vi "Limit Row.vi"(8 "error in (no error)":errorcluster, 10 "Limit File Path":path, 11 "Test Case":string) -> (0 "error out":errorcluster)   [LabVIEW 2024]
doc: "Vi used by the limits configurator to build the limit data."
uses:
  Step Type.ctl
  Numeric Comparison Type.ctl
  String Comparison Type.ctl
  <vilib>/addons/_JKI Toolkits/State Machine/_JKI_lib_State_Machine.llb/Periodic Trigger__ogtk__JKI-SM__jki_lib_state_machine.vi
  <vilib>/addons/_JKI Toolkits/State Machine/_JKI_lib_State_Machine.llb/Select State(s)_err__jki_lib_state_machine.vi
  <vilib>/Utility/file.llb/Read Delimited Spreadsheet (string).vi
  <userlib>/_OpenG.lib/appcontrol/appcontrol.llb/openg_application_control.lvlib
  <vilib>/Utility/file.llb/Write Delimited Spreadsheet (string).vi
panel:
  in  "Comment":string
  in  "Tab Type":enum32{"Numeric", "String", "Boolean", "Action"}(tab)
  in  "Higher Limit":string
  in  "Lower Limit":string
  in  "Numeric Comparison Type":T1 caption="Comparison Type"
  in  "String Comparison Type":T2 caption="Comparison Type"
  in  "Compare String":string
  in  "Boolean Comparison Type":T2 caption="Comparison Type"
  in  "Compare Logic":string(combo)
  out "Title Indicator":string
  in  "Cancel Button":bool
  in  "Add Button":bool
  in  "Step Type":T3
  in  "SubTest Name":string
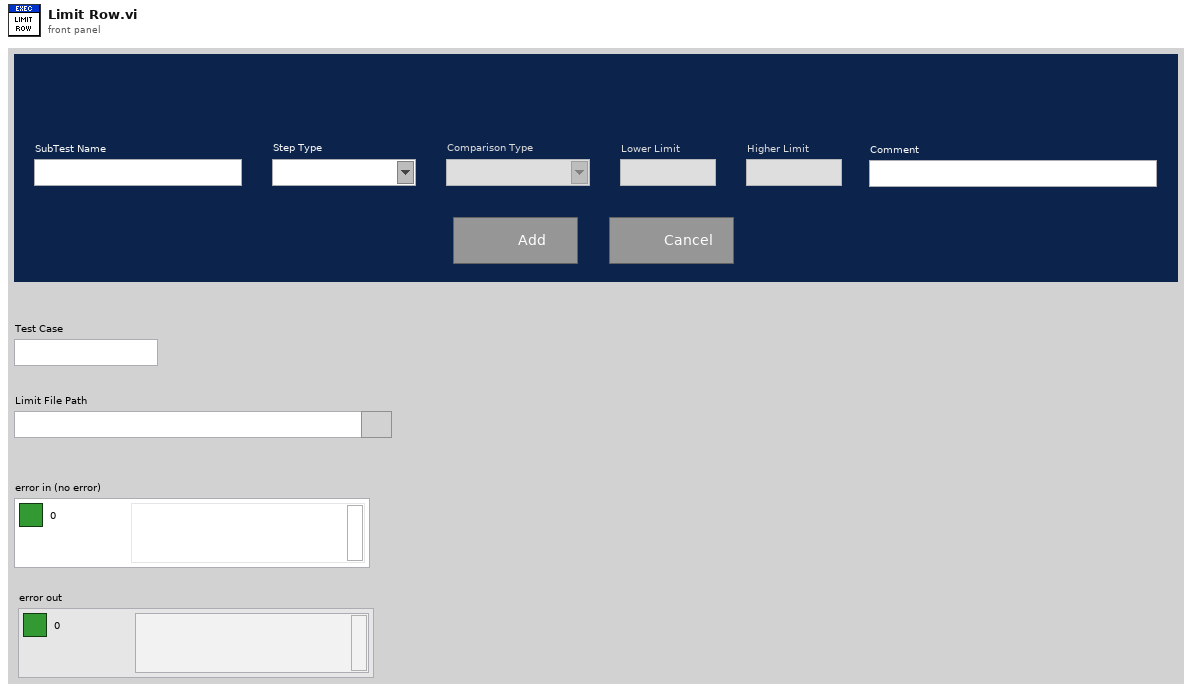
[diagram p1: front panel]
types:
  T1 = typedef "Numeric Comparison Type.ctl" = string
  T2 = typedef "String Comparison Type.ctl" = string
  T3 = typedef "Step Type.ctl" = string
  T4 = enum32{"Invalid", "Standard", "Closed", "Hidden", "Minimized", "Maximized"}
  T5 = enum32{"invalid app kind", "Development System", "Run Time System", "Student Edition", "Embedded LabVIEW", "Evaluation", "Custom"}
  T6 = enum8{"Enabled", "Disabled", "Disabled and Grayed Out"}
  T7 = cluster{"Core":cluster{"Current VI Reference":refnum<vi>, "Close Panel on Exit?":bool}, "Limit Row Array":string[], "Limit File Array":string[][], "Limit File Path":path, "Test Case":string}
  T8 = cluster{"Current VI Reference":refnum<vi>, "Close Panel on Exit?":bool}
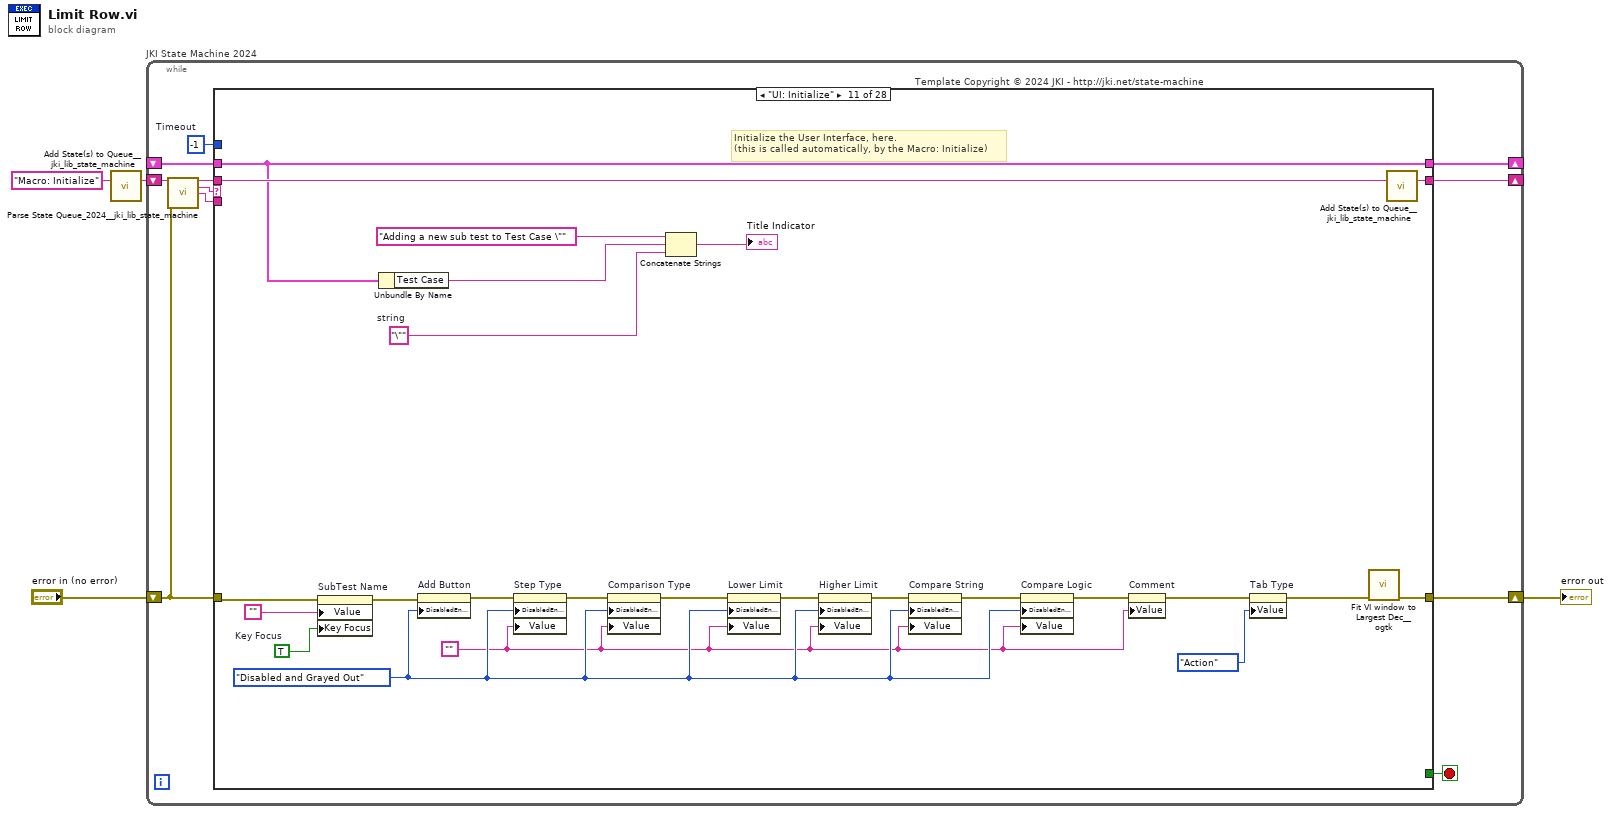
[diagram p0: block diagram]
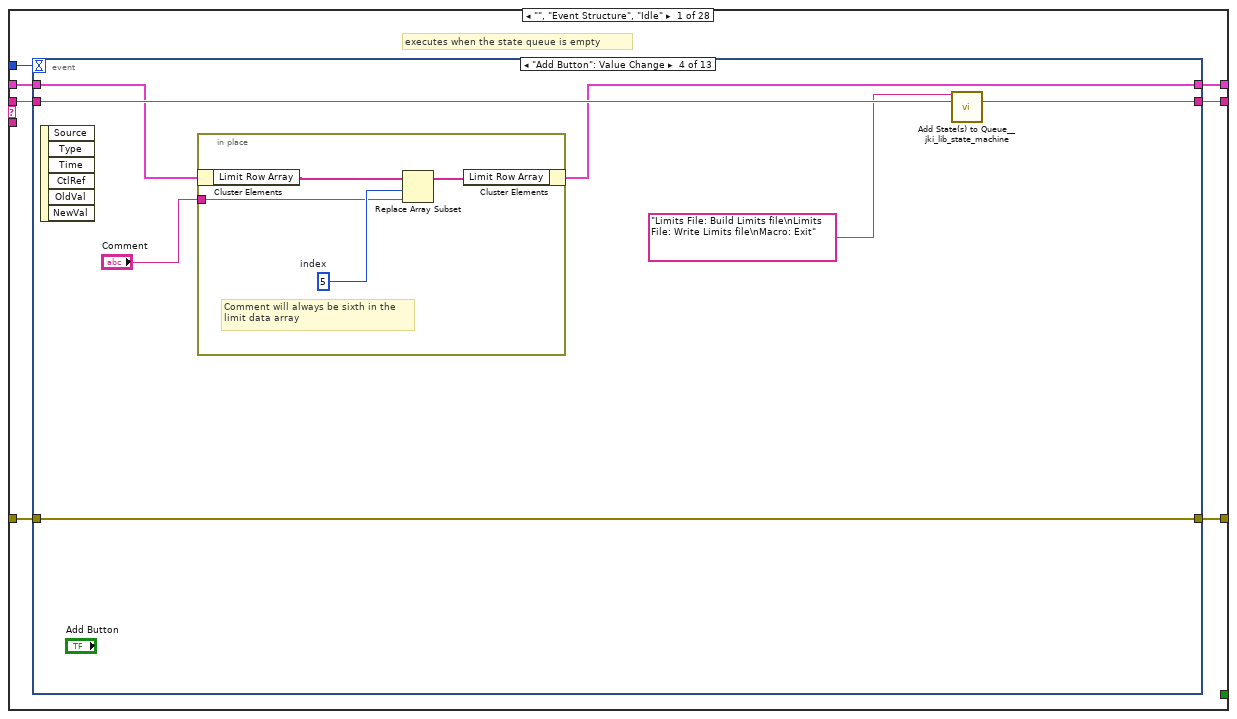
[diagram p2: hidden frame]
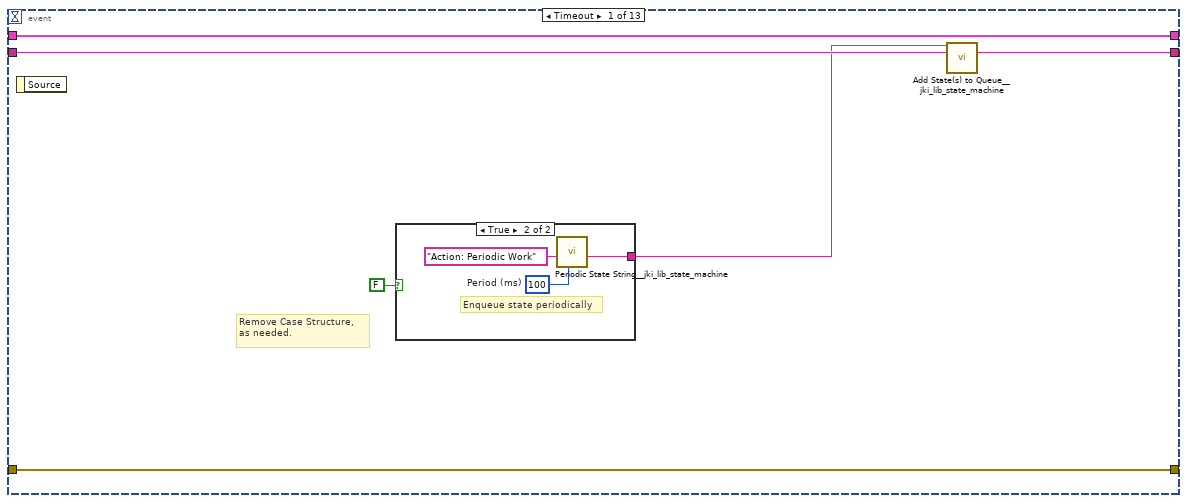
[diagram p3: hidden frame]
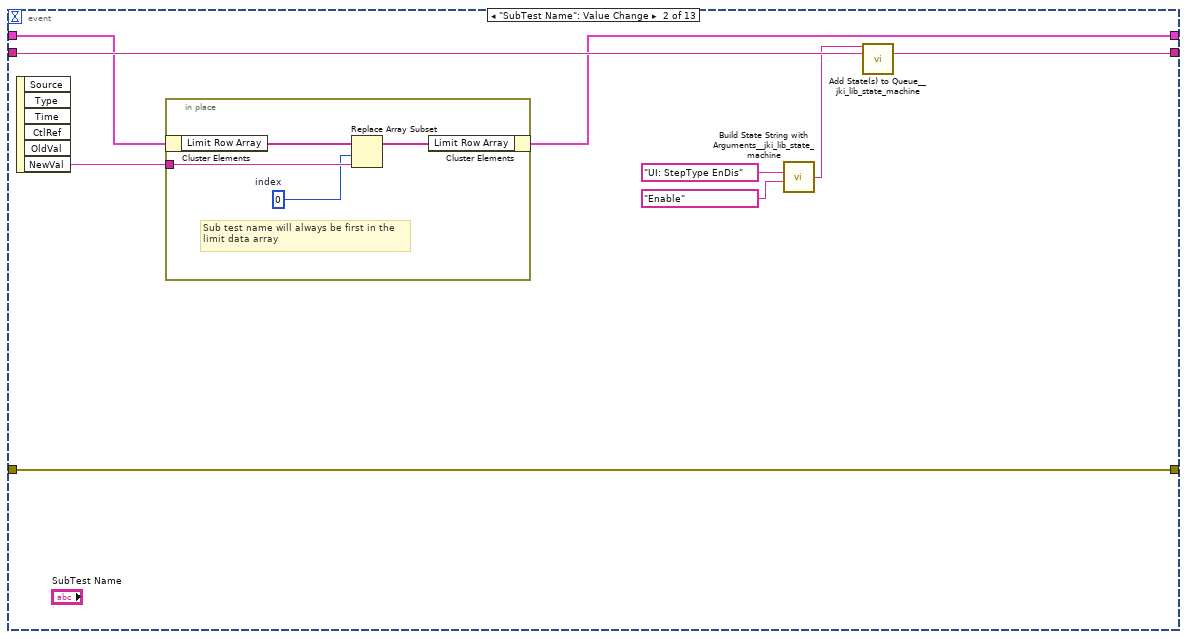
[diagram p5: hidden frame]
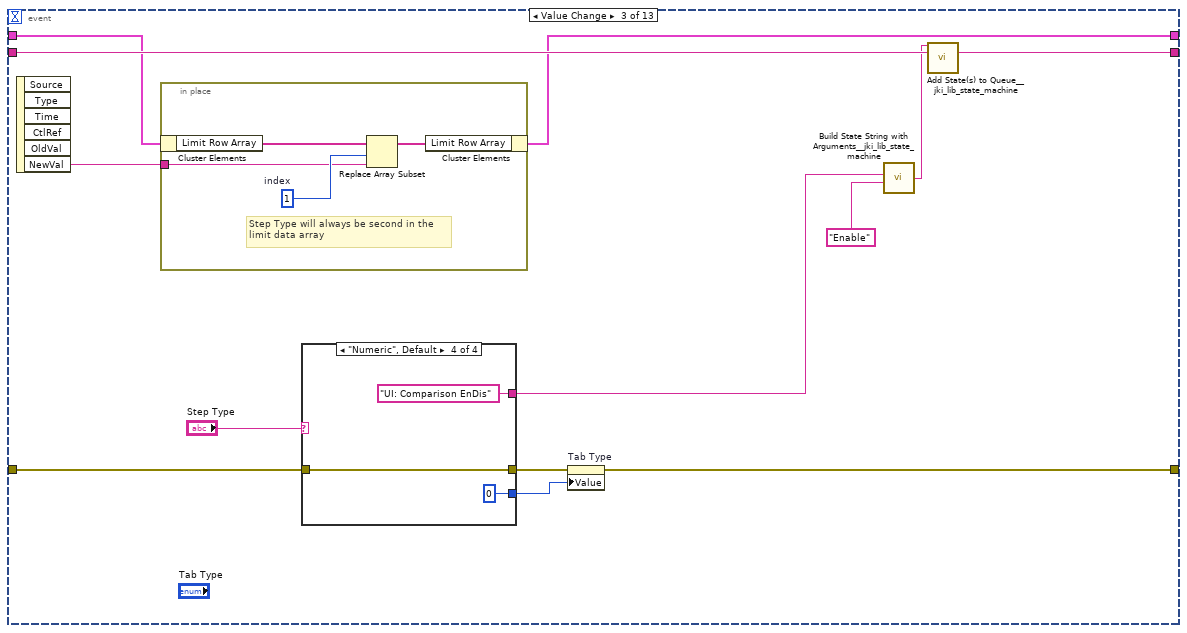
[diagram p6: hidden frame]
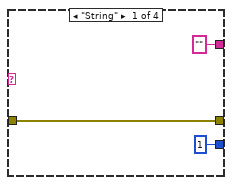
[diagram p7: hidden frame]
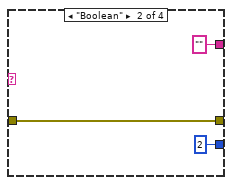
[diagram p8: hidden frame]
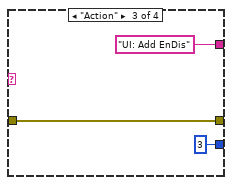
[diagram p9: hidden frame]
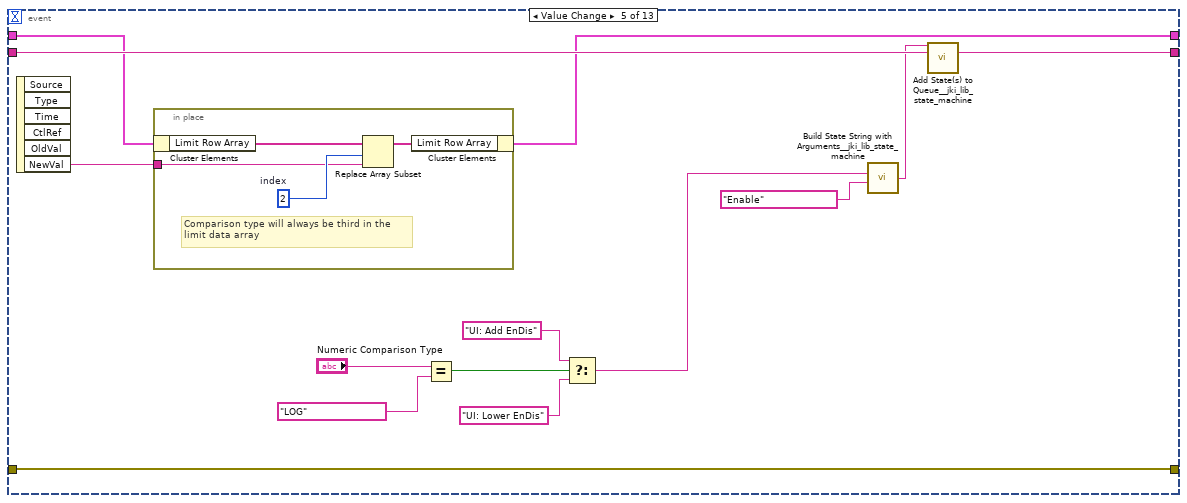
[diagram p10: hidden frame]
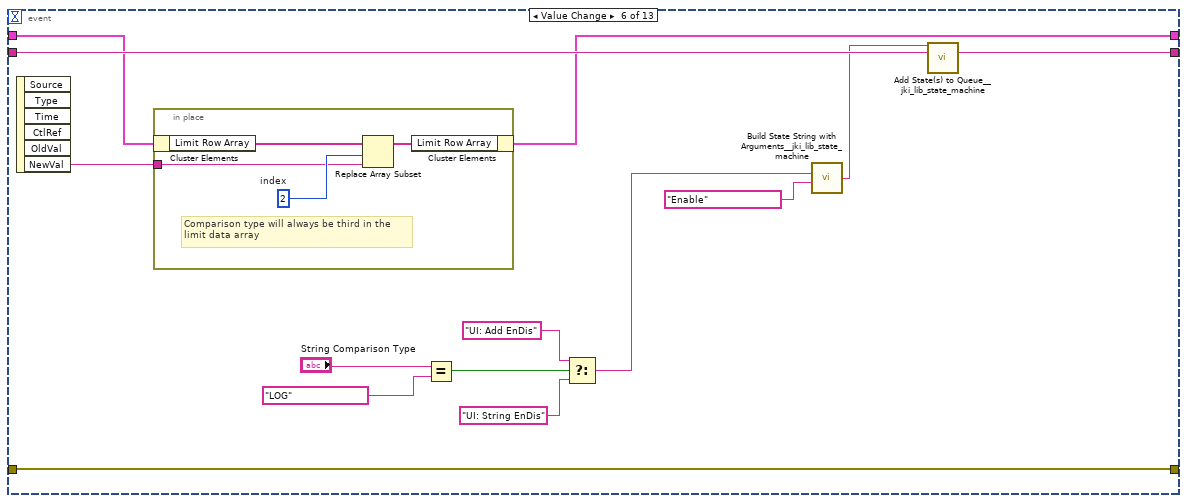
[diagram p11: hidden frame]
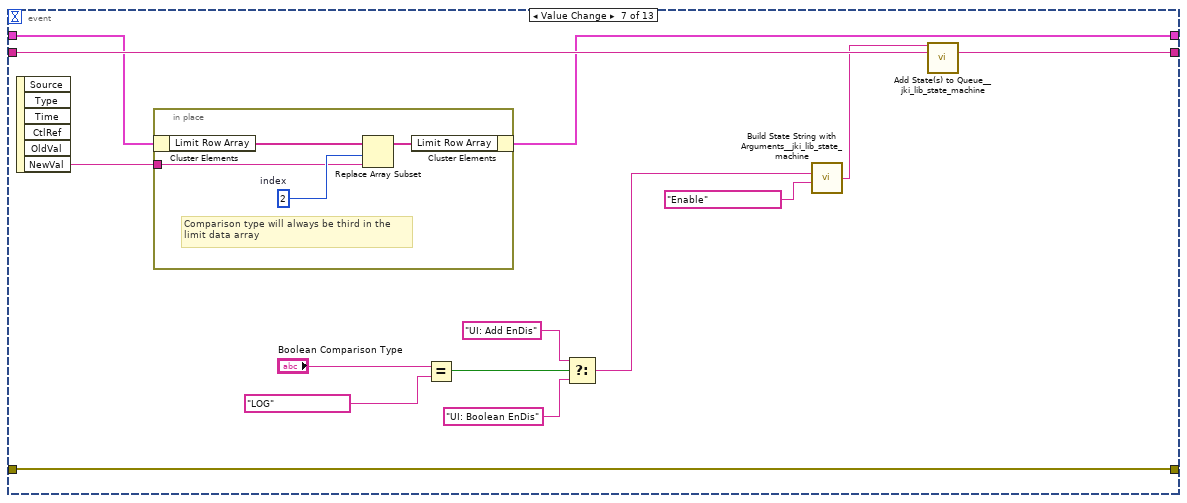
[diagram p12: hidden frame]
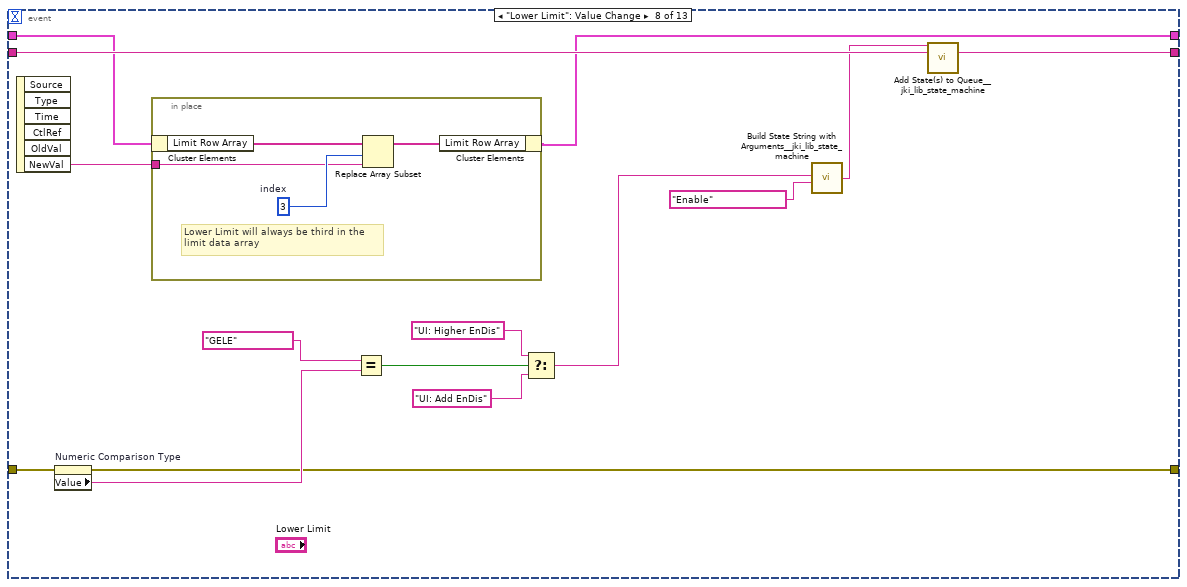
[diagram p13: hidden frame]
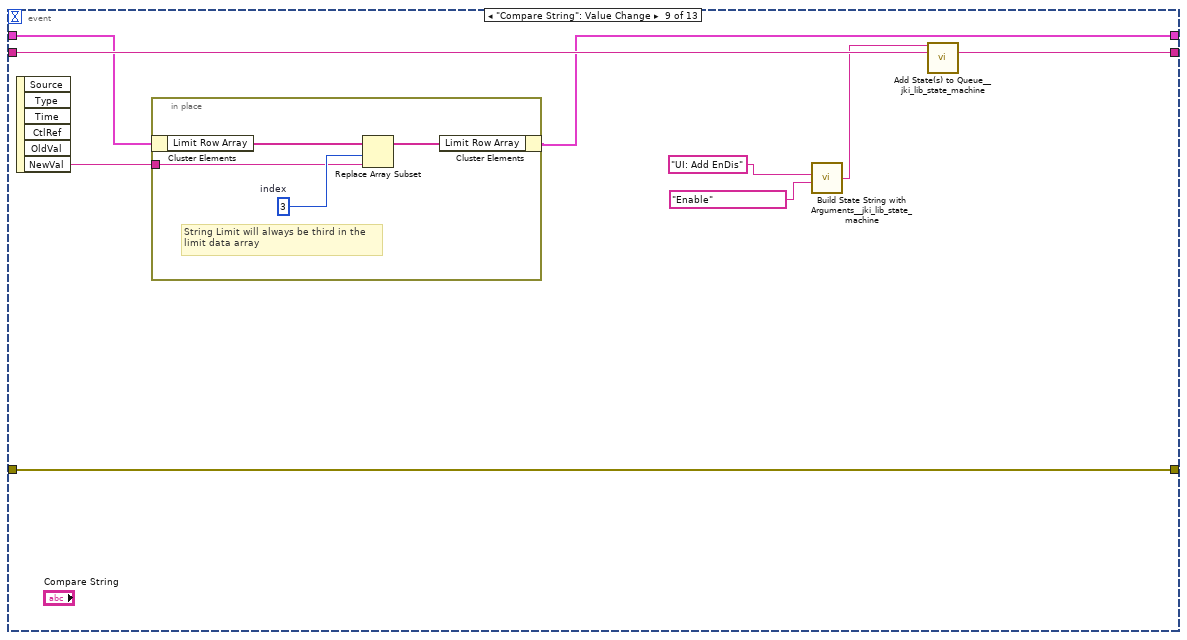
[diagram p14: hidden frame]
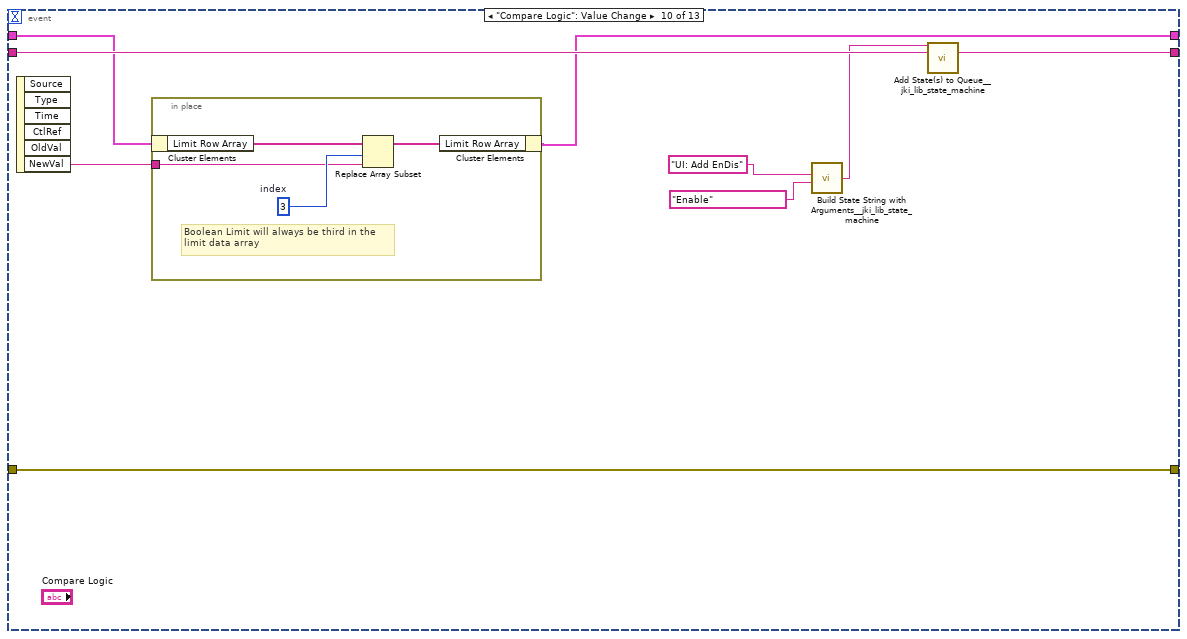
[diagram p15: hidden frame]
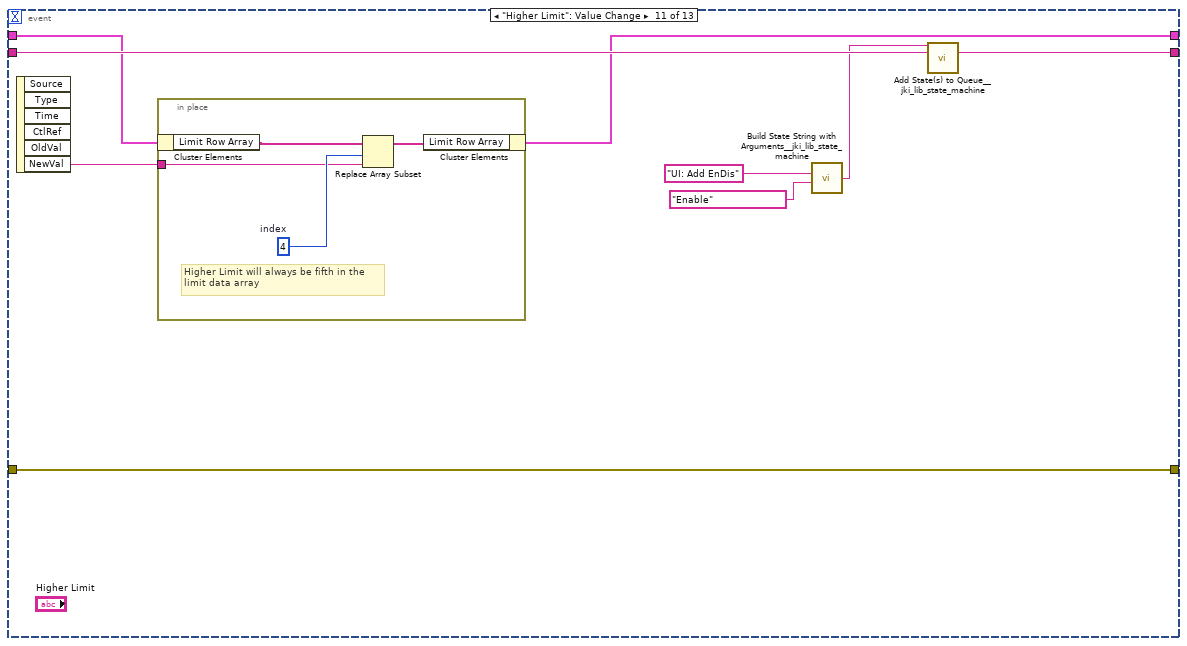
[diagram p16: hidden frame]
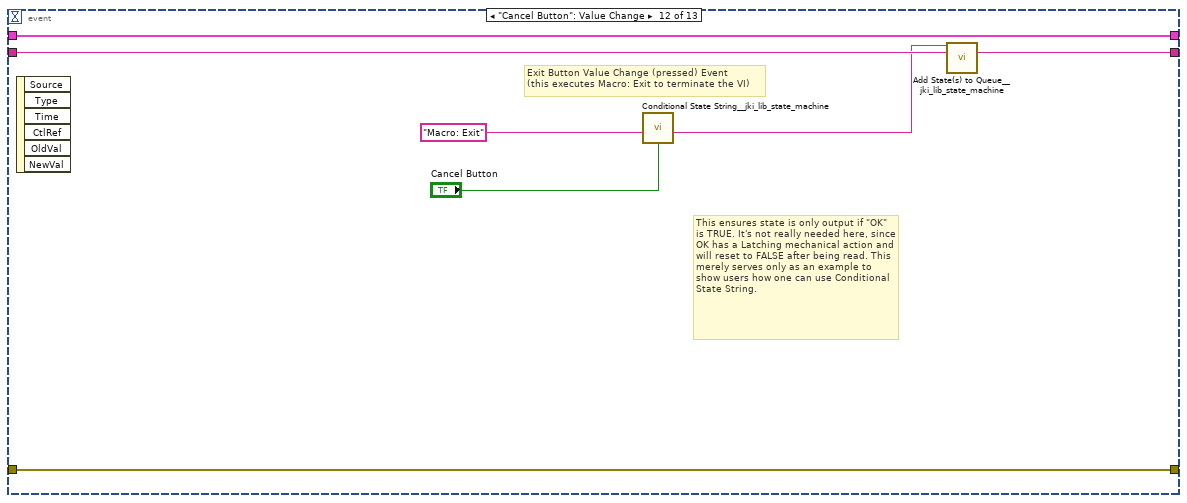
[diagram p17: hidden frame]
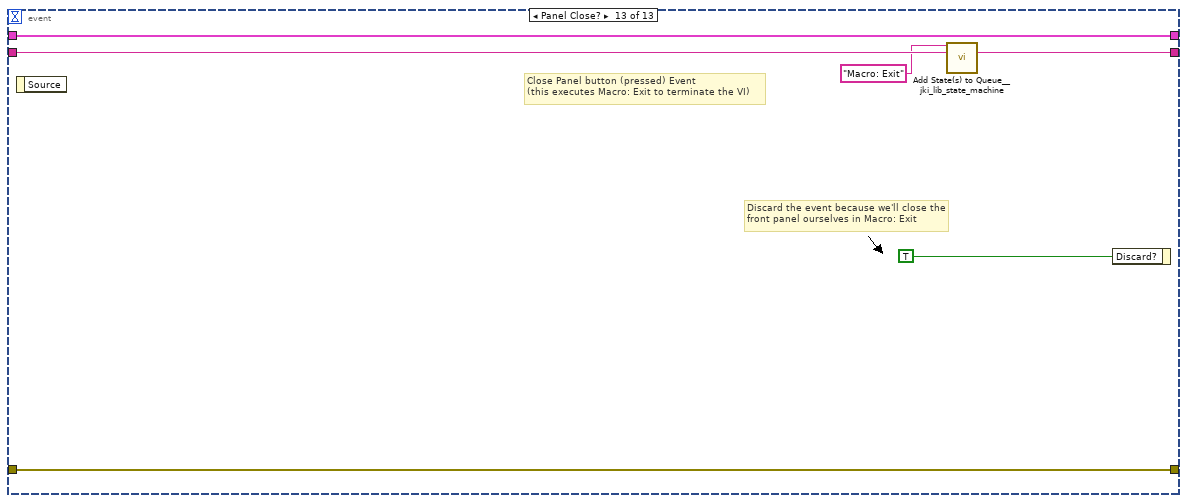
[diagram p18: hidden frame]
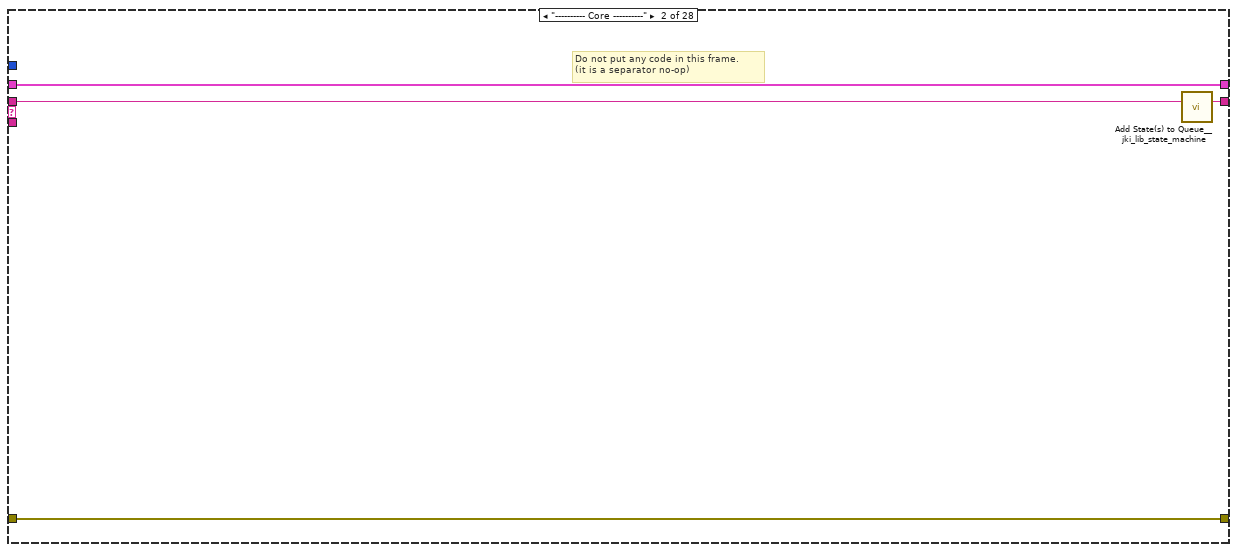
[diagram p19: hidden frame]
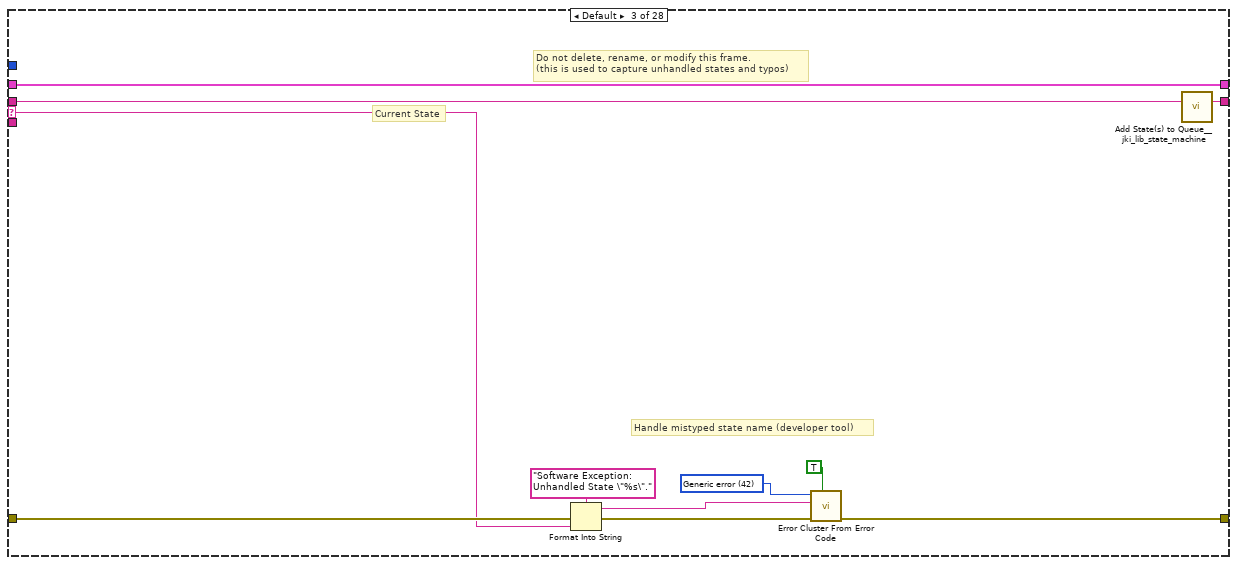
[diagram p20: hidden frame]
diagram:
  n1 = call <vilib>:"Add State(s) to Queue__jki_lib_state_machine.vi"("State(s) in (\"\")"="Macro: Initialize") -> ("States Out"=w4:string)  [unwired: 14 in]
  n2 = while "JKI State Machine 2024" {
    shift-right: [w5] -> _
    shift-left: _ -> [w8]
    shift-right: [w11] -> w1
    shift-left: "error in (no error)" -> [w6]
    shift-right: [w10] -> _
    shift-left: w4 -> [w12]
    stop <- w9 stop-if-true
    w7 = -1  # Timeout
    # "Template Copyright © 2024 JKI - http://jki.net/state-machine"
    n3 = call <vilib>:"Parse State Queue_2024__jki_lib_state_machine.vi"("State Queue"=w12, "Error In (no error)"=w6) -> ("Remaining States"=w14:string, "Current State"=w15:string, "Arguments"=w13:string)  [unwired: 11 in]
    n4 = case shown="\"UI: Initialize\"" w15 {
      selector: w15 -> [_ _ w214 _ _ _ _ _ _ _ _ _ _ _ _ _ _ _ _ _ _ _ _ _ _ _ _ _]
      tunnel: w14 -> [w22 w213 w218 w237 w247 w256 w260 w269 w275 w279 w303 w315 w327 w339 w351 w363 w375 w387 w391 w397 w408 w477 w482 w491 w495 w505 w519 w546]
      tunnel: w13 -> [_ _ _ _ w242 _ _ _ _ _ _ w309 w322 w334 w346 w358 w370 w382 _ w392 w402 _ _ _ _ _ _ _]
      tunnel: w8 -> [w20 w210 w216 w230 w244 w254 w257 _ w270 w276 w293 w313 w325 w337 w349 w361 w373 w385 w389 w395 w404 w474 w479 w489 w492 w499 w512 w544]
      tunnel: [w19 w211 w220 w234 errorcluster {"status"=FALSE, "code"=0, "source"=""} ("error out") w253 w258 w261 w271 w277 w294 w306 w323 w335 w347 w359 w371 w383 w388 w393 w405 w475 w480 w486 w493 w502 w517 w543] -> w11
      tunnel: w6 -> [w16 w211 w219 w234 w243 w253 w258 w261 w272 w277 w296 w307 w324 w336 w348 w360 w372 w384 w388 w394 w406 w475 w480 w486 w493 w503 w517 w542]
      tunnel: [w21 w212 w217 w236 w246 w255 w259 w268 w274 w278 w302 w314 w326 w338 w350 w362 w374 w386 w390 w396 w407 w476 w481 w490 w494 w504 w518 w545] -> w10
      tunnel: [_ _ _ _ _ TRUE _ _ _ _ _ _ _ _ _ _ _ _ _ _ _ _ _ _ _ _ _ _] -> w9
      tunnel: [w18 w210 w216 w235 w244 w254 w257 w267 w270 w276 w293 w313 w325 w337 w349 w361 w373 w385 w389 w395 w404 w474 w479 w489 w492 w501 w511 w544] -> w5
      tunnel: w7 -> [w17 _ _ _ _ _ _ _ _ _ _ _ _ _ _ _ _ _ _ _ _ _ _ _ _ _ _ _]
      frame "", "Event Structure", "Idle" {
        # "executes when the state queue is empty"
        n5 = event shown="[3] \"Add Button\": Value Change" {
          selector: _ -> [_ _ _ _ _ _ _ _ _ _ _ _ _]
          dyn-events: _ -> [_ _ _ _ _ _ _ _ _ _ _ _ _]
          timeout: w17 -> [_ _ _ _ _ _ _ _ _ _ _ _ _]
          tunnel: w22 -> [w28 w39 w54 w78 w95 w113 w131 w150 w163 w176 w188 w203 w209]
          tunnel: [w27 w40 w55 w79 w96 w114 w132 w151 w164 w177 w189 w202 w208] -> w21
          tunnel: w20 -> [w25 w34 w52 w76 w92 w110 w128 w147 w159 w172 w185 w200 w206]
          tunnel: [w26 w35 w47 w80 w93 w111 w129 w139 w161 w174 w186 w201 w207] -> w19
          tunnel: w16 -> [w26 w35 w50 w80 w93 w111 w129 w142 w161 w174 w186 w201 w207]
          tunnel: [w25 w32 w51 w75 w91 w109 w127 w148 w160 w173 w184 w200 w206] -> w18
          event Timeout {
            # "Remove Case Structure, as needed."
            n6 = event-data() -> ()  [unwired: 1 in, 1 out]
            n7 = case shown="True" FALSE {
              tunnel: [_ w31] -> w24
              frame False {
              }
              frame True {
                w29 = u32 100  # Period (ms)
                # "Enqueue state periodically"
                n8 = call <vilib>:"Periodic State String__jki_lib_state_machine.vi"("Period (ms)"=w29, "State"="Action: Periodic Work") -> ("State Out"=w31:string)  [unwired: 9 in]
              }
            }
            n9 = call <vilib>:"Add State(s) to Queue__jki_lib_state_machine.vi"("State(s) in Front (\"\")"=w24, "State(s) in (\"\")"=w28) -> ("States Out"=w27:string)  [unwired: 13 in]
          }
          event "SubTest Name": Value Change {
            n10 = event-data() -> ("NewVal"=w33:string)  [unwired: 1 in, 5 out]
            n11 = in-place {
              in-place-border: w33 -> [w44]
              w42 = 0  # index
              # "Sub test name will always be first in the\nlimit data array"
              n12 = in-place-cluster #1(w34) -> ("Limit Row Array"=w43:string[])
              n13 = Replace Array Subset(array=w43, new element=w44, index=w42) -> (w41:string[])
              n14 = in-place-cluster #1("Limit Row Array"=w41) -> (w32:T7)
            }
            n15 = call <vilib>:"Build State String with Arguments__jki_lib_state_machine.vi"("Arguments (\"\")"="Enable", "State"="UI: StepType EnDis") -> ("State with Arguments"=w36:string)  [unwired: 4 in]
            n16 = call <vilib>:"Add State(s) to Queue__jki_lib_state_machine.vi"("State(s) in Front (\"\")"=w36, "State(s) in (\"\")"=w39) -> ("States Out"=w40:string)  [unwired: 13 in]
          }
          event Value Change {
            n17 = event-data() -> ("NewVal"=w56:T3)  [unwired: 1 in, 5 out]
            n18 = in-place {
              in-place-border: w56 -> [w72]
              w73 = 1  # index
              # "Step Type will always be second in the\nlimit data array"
              n19 = in-place-cluster #2(w52) -> ("Limit Row Array"=w71:string[])
              n20 = Replace Array Subset(array=w71, new element=w72, index=w73) -> (w70:string[])
              n21 = in-place-cluster #2("Limit Row Array"=w70) -> (w51:T7)
            }
            n22 = case shown="\"Numeric\", Default" "Step Type" {
              tunnel: w50 -> [w59 w62 w66 w69]
              tunnel: [w59 w62 w66 w69] -> w48
              tunnel: [1 2 3 0] -> w46
              tunnel: ["" "" "UI: Add EnDis" "UI: Comparison EnDis"] -> w45
              frame "String" {
              }
              frame "Boolean" {
              }
              frame "Action" {
              }
              frame "Numeric", Default {
              }
            }
            n23 = property on="Tab Type" class="TabCtl (strict)"(error in=w48, "Value"=w46) -> (error out=w47:errorcluster)  [unwired: 1 in, 1 out]
            n24 = call <vilib>:"Build State String with Arguments__jki_lib_state_machine.vi"("Arguments (\"\")"="Enable", "State"=w45) -> ("State with Arguments"=w53:string)  [unwired: 4 in]
            n25 = call <vilib>:"Add State(s) to Queue__jki_lib_state_machine.vi"("State(s) in Front (\"\")"=w53, "State(s) in (\"\")"=w54) -> ("States Out"=w55:string)  [unwired: 13 in]
          }
          event "Add Button": Value Change {
            n26 = event-data() -> ()  [unwired: 1 in, 6 out]
            n27 = in-place {
              in-place-border: "Comment" -> [w83]
              w84 = 5  # index
              # "Comment will always be sixth in the\nlimit data array"
              n28 = in-place-cluster #3(w76) -> ("Limit Row Array"=w82:string[])
              n29 = Replace Array Subset(array=w82, new element=w83, index=w84) -> (w81:string[])
              n30 = in-place-cluster #3("Limit Row Array"=w81) -> (w75:T7)
            }
            n31 = call <vilib>:"Add State(s) to Queue__jki_lib_state_machine.vi"("State(s) in Front (\"\")"="Limits File: Build Limits file\nLimits File: Write Limits file\nMacro: Exit", "State(s) in (\"\")"=w78) -> ("States Out"=w79:string)  [unwired: 13 in]
          }
          event Value Change {
            n32 = event-data() -> ("NewVal"=w97:T1)  [unwired: 1 in, 5 out]
            n33 = in-place {
              in-place-border: w97 -> [w101]
              w102 = 2  # index
              # "Comparison type will always be third in the\nlimit data array"
              n34 = in-place-cluster #4(w92) -> ("Limit Row Array"=w100:string[])
              n35 = Replace Array Subset(array=w100, new element=w101, index=w102) -> (w99:string[])
              n36 = in-place-cluster #4("Limit Row Array"=w99) -> (w91:T7)
            }
            n37 = Equal?(x="Numeric Comparison Type", y=T1 "LOG" ("Comparison Type")) -> (x = y?=w88:bool)
            n38 = Select(t="UI: Add EnDis", s=w88, f="UI: Lower EnDis") -> (s? t:f=w85:string)
            n39 = call <vilib>:"Build State String with Arguments__jki_lib_state_machine.vi"("Arguments (\"\")"="Enable", "State"=w85) -> ("State with Arguments"=w94:string)  [unwired: 4 in]
            n40 = call <vilib>:"Add State(s) to Queue__jki_lib_state_machine.vi"("State(s) in Front (\"\")"=w94, "State(s) in (\"\")"=w95) -> ("States Out"=w96:string)  [unwired: 13 in]
          }
          event Value Change {
            n41 = event-data() -> ("NewVal"=w115:T2)  [unwired: 1 in, 5 out]
            n42 = in-place {
              in-place-border: w115 -> [w119]
              w120 = 2  # index
              # "Comparison type will always be third in the\nlimit data array"
              n43 = in-place-cluster #5(w110) -> ("Limit Row Array"=w118:string[])
              n44 = Replace Array Subset(array=w118, new element=w119, index=w120) -> (w117:string[])
              n45 = in-place-cluster #5("Limit Row Array"=w117) -> (w109:T7)
            }
            n46 = Equal?(x="String Comparison Type", y=T2 "LOG" ("String Comparison Type")) -> (x = y?=w108:bool)
            n47 = Select(t="UI: Add EnDis", s=w108, f="UI: String EnDis") -> (s? t:f=w105:string)
            n48 = call <vilib>:"Build State String with Arguments__jki_lib_state_machine.vi"("Arguments (\"\")"="Enable", "State"=w105) -> ("State with Arguments"=w112:string)  [unwired: 4 in]
            n49 = call <vilib>:"Add State(s) to Queue__jki_lib_state_machine.vi"("State(s) in Front (\"\")"=w112, "State(s) in (\"\")"=w113) -> ("States Out"=w114:string)  [unwired: 13 in]
          }
          event Value Change {
            n50 = event-data() -> ("NewVal"=w133:T2)  [unwired: 1 in, 5 out]
            n51 = in-place {
              in-place-border: w133 -> [w137]
              w138 = 2  # index
              # "Comparison type will always be third in the\nlimit data array"
              n52 = in-place-cluster #6(w128) -> ("Limit Row Array"=w136:string[])
              n53 = Replace Array Subset(array=w136, new element=w137, index=w138) -> (w135:string[])
              n54 = in-place-cluster #6("Limit Row Array"=w135) -> (w127:T7)
            }
            n55 = Equal?(x="Boolean Comparison Type", y=T2 "LOG" ("Boolean Comparison Type")) -> (x = y?=w126:bool)
            n56 = Select(t="UI: Add EnDis", s=w126, f="UI: Boolean EnDis") -> (s? t:f=w123:string)
            n57 = call <vilib>:"Build State String with Arguments__jki_lib_state_machine.vi"("Arguments (\"\")"="Enable", "State"=w123) -> ("State with Arguments"=w130:string)  [unwired: 4 in]
            n58 = call <vilib>:"Add State(s) to Queue__jki_lib_state_machine.vi"("State(s) in Front (\"\")"=w130, "State(s) in (\"\")"=w131) -> ("States Out"=w132:string)  [unwired: 13 in]
          }
          event "Lower Limit": Value Change {
            n59 = event-data() -> ("NewVal"=w152:string)  [unwired: 1 in, 5 out]
            n60 = property on="Numeric Comparison Type" class="CmbBox (strict)"(error in=w142) -> (error out=w139:errorcluster, "Value"=w141:T1)  [unwired: 1 in, 1 out]
            n61 = in-place {
              in-place-border: w152 -> [w156]
              w157 = 3  # index
              # "Lower Limit will always be third in the\nlimit data array"
              n62 = in-place-cluster #7(w147) -> ("Limit Row Array"=w155:string[])
              n63 = Replace Array Subset(array=w155, new element=w156, index=w157) -> (w154:string[])
              n64 = in-place-cluster #7("Limit Row Array"=w154) -> (w148:T7)
            }
            n65 = Equal?(x=T1 "GELE" ("Numeric Comparison Type"), y=w141) -> (x = y?=w146:bool)
            n66 = Select(t="UI: Higher EnDis", s=w146, f="UI: Add EnDis") -> (s? t:f=w143:string)
            n67 = call <vilib>:"Build State String with Arguments__jki_lib_state_machine.vi"("Arguments (\"\")"="Enable", "State"=w143) -> ("State with Arguments"=w149:string)  [unwired: 4 in]
            n68 = call <vilib>:"Add State(s) to Queue__jki_lib_state_machine.vi"("State(s) in Front (\"\")"=w149, "State(s) in (\"\")"=w150) -> ("States Out"=w151:string)  [unwired: 13 in]
          }
          event "Compare String": Value Change {
            n69 = event-data() -> ("NewVal"=w165:string)  [unwired: 1 in, 5 out]
            n70 = in-place {
              in-place-border: w165 -> [w169]
              w170 = 3  # index
              # "String Limit will always be third in the\nlimit data array"
              n71 = in-place-cluster #8(w159) -> ("Limit Row Array"=w168:string[])
              n72 = Replace Array Subset(array=w168, new element=w169, index=w170) -> (w167:string[])
              n73 = in-place-cluster #8("Limit Row Array"=w167) -> (w160:T7)
            }
            n74 = call <vilib>:"Build State String with Arguments__jki_lib_state_machine.vi"("Arguments (\"\")"="Enable", "State"="UI: Add EnDis") -> ("State with Arguments"=w162:string)  [unwired: 4 in]
            n75 = call <vilib>:"Add State(s) to Queue__jki_lib_state_machine.vi"("State(s) in Front (\"\")"=w162, "State(s) in (\"\")"=w163) -> ("States Out"=w164:string)  [unwired: 13 in]
          }
          event "Compare Logic": Value Change {
            n76 = event-data() -> ("NewVal"=w178:string)  [unwired: 1 in, 5 out]
            n77 = in-place {
              in-place-border: w178 -> [w182]
              w183 = 3  # index
              # "Boolean Limit will always be third in the\nlimit data array"
              n78 = in-place-cluster #9(w172) -> ("Limit Row Array"=w181:string[])
              n79 = Replace Array Subset(array=w181, new element=w182, index=w183) -> (w180:string[])
              n80 = in-place-cluster #9("Limit Row Array"=w180) -> (w173:T7)
            }
            n81 = call <vilib>:"Build State String with Arguments__jki_lib_state_machine.vi"("Arguments (\"\")"="Enable", "State"="UI: Add EnDis") -> ("State with Arguments"=w175:string)  [unwired: 4 in]
            n82 = call <vilib>:"Add State(s) to Queue__jki_lib_state_machine.vi"("State(s) in Front (\"\")"=w175, "State(s) in (\"\")"=w176) -> ("States Out"=w177:string)  [unwired: 13 in]
          }
          event "Higher Limit": Value Change {
            n83 = event-data() -> ("NewVal"=w190:string)  [unwired: 1 in, 5 out]
            n84 = in-place {
              in-place-border: w190 -> [w195]
              w196 = 4  # index
              # "Higher Limit will always be fifth in the\nlimit data array"
              n85 = in-place-cluster #10(w185) -> ("Limit Row Array"=w194:string[])
              n86 = Replace Array Subset(array=w194, new element=w195, index=w196) -> (w193:string[])
              n87 = in-place-cluster #10("Limit Row Array"=w193) -> (w184:T7)
            }
            n88 = call <vilib>:"Build State String with Arguments__jki_lib_state_machine.vi"("Arguments (\"\")"="Enable", "State"="UI: Add EnDis") -> ("State with Arguments"=w187:string)  [unwired: 4 in]
            n89 = call <vilib>:"Add State(s) to Queue__jki_lib_state_machine.vi"("State(s) in Front (\"\")"=w187, "State(s) in (\"\")"=w188) -> ("States Out"=w189:string)  [unwired: 13 in]
          }
          event "Cancel Button": Value Change {
            # "This ensures state is only output if \"OK\" is TRUE. It's not really needed here, since OK has a Latching mechanical action and will reset to FALSE after being read. This merely serves only as an example to show users how one can use Conditional State String."
            # "Exit Button Value Change (pressed) Event\n(this executes Macro: Exit to terminate the VI)"
            n90 = event-data() -> ()  [unwired: 1 in, 6 out]
            n91 = call <vilib>:"Conditional State String__jki_lib_state_machine.vi"("Do State(s)?"="Cancel Button", "State"="Macro: Exit") -> ("State Out"=w198:string)  [unwired: 7 in]
            n92 = call <vilib>:"Add State(s) to Queue__jki_lib_state_machine.vi"("State(s) in Front (\"\")"=w198, "State(s) in (\"\")"=w203) -> ("States Out"=w202:string)  [unwired: 13 in]
          }
          event Panel Close? {
            # "Discard the event because we'll close the front panel ourselves in Macro: Exit"
            # "Close Panel button (pressed) Event\n(this executes Macro: Exit to terminate the VI)"
            n93 = event-data() -> ()  [unwired: 1 in, 1 out]
            n94 = call <vilib>:"Add State(s) to Queue__jki_lib_state_machine.vi"("State(s) in Front (\"\")"="Macro: Exit", "State(s) in (\"\")"=w209) -> ("States Out"=w208:string)  [unwired: 13 in]
            n95 = event-data("Discard?"=TRUE) -> ()  [unwired: 1 in, 1 out]
          }
        }
      }
      frame "---------- Core ----------" {
        # "Do not put any code in this frame.\n(it is a separator no-op)"
        n96 = call <vilib>:"Add State(s) to Queue__jki_lib_state_machine.vi"("State(s) in (\"\")"=w213) -> ("States Out"=w212:string)  [unwired: 14 in]
      }
      frame Default {
        w223 = 42 items=["No error", "Argument error", "Memory is full", "Out of zone", "End of file", "File already open", "Generic file I/O error", "File not found", "File permission error", "Disk is full", "Duplicate path", "Too many files open", "System feature not enabled", "Resource file not found", "Cannot add resource", "Resource not found", "Image not found", "Image memory error", "Pen does not exist", "Config type invalid", "Config token not found", "Config parse error", "Config memory error", "Bad external code format", "Bad external code offset", "External code not present", "Null window", "Destroy window error", "Null menu", "Print aborted", "Bad print record", "Print driver error", "Windows error during printing", "Memory error during printing", "Print dialog error", "Generic print error", "Invalid device refnum", "Device not found", "Device parameter error", "Device unit error", "Cannot open device", "Device call aborted", "Generic error", "Cancelled by user", "Object ID too low", "Object ID too high", "Object not in heap", "Unknown heap", "Unknown object (invalid DefProc)", "Unknown object (DefProc not in table)", "Message out of range", "Invalid (null) method", "Unknown message", "Manager call not supported", "Bad address", "Network operation in progress", "Network operation timed out", "Connection is busy", "Network attribute not supported", "Network error", "Address in use", "System out of memory", "Connection aborted", "Connection refused", "Not connected", "Already connected", "Connection closed", "Initialization error (interapplication manager)", "Bad occurrence", "Wait on unbound occurrence handler", "Occurrence queue overflow", "Datalog type conflict", "Unused", "Unrecognized type (interapplication manager)", "Memory corrupt", "Failed to make temporary DLL", "Old CIN version", "Drag socket not found", "Failed to load drop-object", "Failed to register OLE object", "Failed to release OLE object", "Format specifier type mismatch", "Unknown format specifier", "Too few format specifiers", "Too many format specifiers", "Scan failed", "Newer CIN version", "Error converting to variant", "Runtime menu error", "Password tampered", "Variant attribute not found", "Incompatible variant data type", "Event data is not available", "Event Store is not present", "Occurrence is not found", "Event Queue is not created", "Event info is not available", "Refnum passed is NULL", "Error retrieving Class GUID", "Error retrieving CoClass GUID", "Error retrieving TypeLib GUID.", "Bad built application magic bytes.", "Specific driver is different from the specific driver associated with the Logical Name.", "There is no session opened to the class driver.", "Max Error", "MAX - Error with config objects", "MAX - Error loading configuration", "MAX - Group not supported"]
        # "Current State"
        # "Do not delete, rename, or modify this frame.\n(this is used to capture unhandled states and typos)"
        # "Handle mistyped state name (developer tool)"
        n97 = Format Into String(format string="Software Exception: Unhandled State \"%s\"." ("message"), error in=w219, w214) -> (resulting string=w222:string, error out=w221:errorcluster)  [unwired: 1 in]
        n98 = call <vilib>:"Error Cluster From Error Code.vi"("show call chain? (False)"=TRUE, "error in (no error)"=w221, "error message (\"\")"=w222, "error code (0)"=w223) -> ("error out"=w220:errorcluster)  [unwired: 5 in]
        n99 = call <vilib>:"Add State(s) to Queue__jki_lib_state_machine.vi"("State(s) in (\"\")"=w218) -> ("States Out"=w217:string)  [unwired: 14 in]
      }
      frame "Initialize Core Data" {
        # "Do not delete, rename, or modify this frame.\n(this is used to determine panel behavior on exit)"
        # "originally closed?"
        # "exe?"
        # "If panel starts closed or is an EXE, then close it when we exit"
        n100 = property class="VI"() -> ("FP.State"=w227:T4)  [unwired: 2 in, 2 out]
        n101 = property class="App"() -> ("App.Kind"=w233:T5)  [unwired: 2 in, 2 out]
        n102 = control-ref of="Current VI Reference"() -> (w228:refnum<vi>)
        n103 = Equal?(x=w227, y=T4."Closed" ("Front Panel Window:State")) -> (x = y?=w225:bool)
        n104 = Equal?(x=w233, y=T5."Run Time System" ("Application:Kind")) -> (x = y?=w231:bool)
        n105 = Or(x=w225, y=w231) -> (x .or. y?=w229:bool)
        n106 = Bundle By Name(cluster=w230, "Core.Current VI Reference"=w228, "Core.Close Panel on Exit?"=w229) -> (w235:T7)
        n107 = call <vilib>:"Add State(s) to Queue__jki_lib_state_machine.vi"("State(s) in (\"\")"=w237) -> ("States Out"=w236:string)  [unwired: 14 in]
      }
      frame "Error Handler" {
        # "When running as sourcecode, this function will add previous state data to the error message to aid the developer in troubleshoot errors.\nIf run as an executable, no additional information is added to the error message."
        # "This state receives both Errors and Warnings which is how the Status of this wire can be FALSE"
        # "Unhandled Error -- Display it"
        # "Handle any errors or warnings here.\nYou can also output any states to clean-up after errors or warnings occur"
        # "Clear error or warning"
        n108 = disable-structure shown="Default" {
          disable-tunnel: w243 -> [w250 w251]
          disable-tunnel: w242 -> [w249 _]
          disable-tunnel: [w248 w251] -> w241
          frame condition #0 (active) {
            n109 = call <vilib>:"Append Error Details__jki_lib_state_machine.vi"("error in (no error)"=w250, "Previous State and Argument(s)"=w249) -> ("error out"=w248:errorcluster)  [unwired: 9 in]
          }
          frame condition #1 {
          }
        }
        n110 = call <vilib>:"General Error Handler.vi"("error in (no error)"=w241) -> ()  [unwired: 10 in, 5 out]
        n111 = call-poly <vilib>:"Select State(s)__jki_lib_state_machine.vi"("State(s) if True (\"\")"="/* Post Error States", "Select"=w241, "State(s) if False (\"\")"="/* Post Warning States") -> ("States Out"=w239:string)  [unwired: 12 in]
        n112 = call <vilib>:"Add State(s) to Queue__jki_lib_state_machine.vi"("State(s) in Front (\"\")"=w239, "State(s) in (\"\")"=w247) -> ("States Out"=w246:string)  [unwired: 13 in]
      }
      frame "Exit" {
        # "Do not put any code in this frame.\n(No errors that occur here will be handled.)"
        n113 = call <vilib>:"Add State(s) to Queue__jki_lib_state_machine.vi"("State(s) in (\"\")"=w256) -> ("States Out"=w255:string)  [unwired: 14 in]
      }
      frame "---------- Data ----------" {
        # "Do not put any code in this frame.\n(It is a separator no-op. You can make a copy of this frame to create a new Data frame)"
        n114 = call <vilib>:"Add State(s) to Queue__jki_lib_state_machine.vi"("State(s) in (\"\")"=w260) -> ("States Out"=w259:string)  [unwired: 14 in]
      }
      frame "Data: Initialize" {
        w264 = string[][] []  # Limit File Array
        w265 = string[] [" ", " ", " ", " ", " ", ""]  # Limit Row Array
        w266 = T8 {"Current VI Reference"=refnum, "Close Panel on Exit?"=FALSE}  # Core
        # "Data names and types of shift register data are defined by this bundle."
        # "Initialize the shift-register data, here.\n(data names are defined by what you wire into the bundle function)"
        n115 = Bundle("Core"=w266, "Limit Row Array"=w265, "Limit File Array"=w264, "Limit File Path"="Limit File Path", "Test Case"="Test Case") -> (w267:T7)  [unwired: 1 in]
        n116 = call <vilib>:"Add State(s) to Queue__jki_lib_state_machine.vi"("State(s) in (\"\")"=w269) -> ("States Out"=w268:string)  [unwired: 14 in]
      }
      frame "Data: Cleanup" {
        # "Cleanup any data and references, here.\n(this is called automatically, by the Macro: Exit)"
        n117 = Unbundle By Name(w270) -> ("Core.Current VI Reference"=w273:refnum<vi>)
        n118 = Close Reference(reference=w273, error in (no error)=w272) -> (error out=w271:errorcluster)
        n119 = call <vilib>:"Add State(s) to Queue__jki_lib_state_machine.vi"("State(s) in (\"\")"=w275) -> ("States Out"=w274:string)  [unwired: 14 in]
      }
      frame "---------- UI ----------" {
        # "Do not put any code in this frame.\n(It is a separator no-op. You can make a copy of this frame to create a new UI frame)"
        n120 = call <vilib>:"Add State(s) to Queue__jki_lib_state_machine.vi"("State(s) in (\"\")"=w279) -> ("States Out"=w278:string)  [unwired: 14 in]
      }
      frame "UI: Initialize" {
        w288 = TRUE  # Key Focus
        w290 = "\""  # string
        w280 = ""
        w283 = T6."Disabled and Grayed Out" ("Disabled")
        # "Initialize the User Interface, here.\n(this is called automatically, by the Macro: Initialize)"
        n121 = property on="SubTest Name" class="Str"(error in=w296, "Value"="" ("SubTest Name"), "Key Focus"=w288) -> (error out=w297:errorcluster)  [unwired: 1 in, 1 out]
        n122 = Unbundle By Name(w293) -> ("Test Case"=w291:string)
        n123 = property on="Add Button" class="Bool"(error in=w297, "DisabledEnum"=w283) -> (error out=w301:errorcluster)  [unwired: 1 in, 1 out]
        n124 = property on="Step Type" class="CmbBox (strict)"(error in=w301, "DisabledEnum"=w283, "Value"=w280) -> (error out=w300:errorcluster)  [unwired: 1 in, 1 out]
        n125 = property on="Comparison Type" class="CmbBox (strict)"(error in=w300, "DisabledEnum"=w283, "Value"=w280) -> (error out=w299:errorcluster)  [unwired: 1 in, 1 out]
        n126 = Concatenate Strings("Adding a new sub test to Test Case \"", w291, w290) -> (→"Title Indicator":string)
        n127 = property on="Lower Limit" class="Str"(error in=w299, "DisabledEnum"=w283, "Value"=w280) -> (error out=w298:errorcluster)  [unwired: 1 in, 1 out]
        n128 = property on="Higher Limit" class="Str"(error in=w298, "DisabledEnum"=w283, "Value"=w280) -> (error out=w287:errorcluster)  [unwired: 1 in, 1 out]
        n129 = property on="Compare String" class="Str"(error in=w287, "DisabledEnum"=w283, "Value"=w280) -> (error out=w284:errorcluster)  [unwired: 1 in, 1 out]
        n130 = property on="Compare Logic" class="CmbBox"(error in=w284, "DisabledEnum"=w283, "Value"=w280) -> (error out=w282:errorcluster)  [unwired: 1 in, 1 out]
        n131 = property on="Comment" class="Str"(error in=w282, "Value"=w280) -> (error out=w281:errorcluster)  [unwired: 1 in, 1 out]
        n132 = property on="Tab Type" class="TabCtl (strict)"(error in=w281, "Value"=enum32{"Numeric", "String", "Boolean", "Action"}."Action" ("Tab Type")) -> (error out=w286:errorcluster)  [unwired: 1 in, 1 out]
        n133 = call <userlib>:"Fit VI window to Largest Dec__ogtk.vi"("error in (no error)"=w286) -> ("error out"=w294:errorcluster)  [unwired: 5 in, 1 out]
        n134 = call <vilib>:"Add State(s) to Queue__jki_lib_state_machine.vi"("State(s) in (\"\")"=w303) -> ("States Out"=w302:string)  [unwired: 14 in]
      }
      frame "UI: Comparison EnDis" {
        # "Initialize the User Interface, here.\n(this is called automatically, by the Macro: Initialize)"
        n135 = Equal?(x=w309, y="Disable") -> (x = y?=w305:bool)
        n136 = Not(x=w305) -> (.not. x?=w304:bool)
        n137 = Select(t=T6."Disabled and Grayed Out" ("Disabled"), s=w305, f=T6."Enabled" ("Disabled")) -> (s? t:f=w308:T6)
        n138 = property on="Comparison Type" class="CmbBox (strict)"(error in=w307, "DisabledEnum"=w308, "Key Focus"=w304) -> (error out=w306:errorcluster)  [unwired: 1 in, 1 out]
        n139 = call <vilib>:"Add State(s) to Queue__jki_lib_state_machine.vi"("State(s) in (\"\")"=w315) -> ("States Out"=w314:string)  [unwired: 14 in]
      }
      frame "UI: StepType EnDis" {
        # "Initialize the User Interface, here.\n(this is called automatically, by the Macro: Initialize)"
        n140 = Equal?(x=w322, y="Disable") -> (x = y?=w317:bool)
        n141 = Not(x=w317) -> (.not. x?=w316:bool)
        n142 = Select(t=T6."Disabled and Grayed Out" ("Disabled"), s=w317, f=T6."Enabled" ("Disabled")) -> (s? t:f=w318:T6)
        n143 = property on="Step Type" class="CmbBox (strict)"(error in=w324, "DisabledEnum"=w318, "Key Focus"=w316) -> (error out=w323:errorcluster)  [unwired: 1 in, 1 out]
        n144 = call <vilib>:"Add State(s) to Queue__jki_lib_state_machine.vi"("State(s) in (\"\")"=w327) -> ("States Out"=w326:string)  [unwired: 14 in]
      }
      frame "UI: Lower EnDis" {
        # "Initialize the User Interface, here.\n(this is called automatically, by the Macro: Initialize)"
        n145 = Equal?(x=w334, y="Disable") -> (x = y?=w329:bool)
        n146 = Not(x=w329) -> (.not. x?=w328:bool)
        n147 = Select(t=T6."Disabled and Grayed Out" ("Disabled"), s=w329, f=T6."Enabled" ("Disabled")) -> (s? t:f=w330:T6)
        n148 = property on="Lower Limit" class="Str"(error in=w336, "DisabledEnum"=w330, "Key Focus"=w328) -> (error out=w335:errorcluster)  [unwired: 1 in, 1 out]
        n149 = call <vilib>:"Add State(s) to Queue__jki_lib_state_machine.vi"("State(s) in (\"\")"=w339) -> ("States Out"=w338:string)  [unwired: 14 in]
      }
      frame "UI: Higher EnDis" {
        # "Initialize the User Interface, here.\n(this is called automatically, by the Macro: Initialize)"
        n150 = Equal?(x=w346, y="Disable") -> (x = y?=w341:bool)
        n151 = Not(x=w341) -> (.not. x?=w340:bool)
        n152 = Select(t=T6."Disabled and Grayed Out" ("Disabled"), s=w341, f=T6."Enabled" ("Disabled")) -> (s? t:f=w342:T6)
        n153 = property on="Higher Limit" class="Str"(error in=w348, "DisabledEnum"=w342, "Key Focus"=w340) -> (error out=w347:errorcluster)  [unwired: 1 in, 1 out]
        n154 = call <vilib>:"Add State(s) to Queue__jki_lib_state_machine.vi"("State(s) in (\"\")"=w351) -> ("States Out"=w350:string)  [unwired: 14 in]
      }
      frame "UI: Add EnDis" {
        # "Initialize the User Interface, here.\n(this is called automatically, by the Macro: Initialize)"
        n155 = Equal?(x=w358, y="Disable") -> (x = y?=w353:bool)
        n156 = Not(x=w353) -> (.not. x?=w352:bool)
        n157 = Select(t=T6."Disabled and Grayed Out" ("Disabled"), s=w353, f=T6."Enabled" ("Disabled")) -> (s? t:f=w354:T6)
        n158 = property on="Add Button" class="Bool"(error in=w360, "DisabledEnum"=w354, "Key Focus"=w352) -> (error out=w359:errorcluster)  [unwired: 1 in, 1 out]
        n159 = call <vilib>:"Add State(s) to Queue__jki_lib_state_machine.vi"("State(s) in (\"\")"=w363) -> ("States Out"=w362:string)  [unwired: 14 in]
      }
      frame "UI: String EnDis" {
        # "Initialize the User Interface, here.\n(this is called automatically, by the Macro: Initialize)"
        n160 = Equal?(x=w370, y="Disable") -> (x = y?=w365:bool)
        n161 = Not(x=w365) -> (.not. x?=w364:bool)
        n162 = Select(t=T6."Disabled and Grayed Out" ("Disabled"), s=w365, f=T6."Enabled" ("Disabled")) -> (s? t:f=w366:T6)
        n163 = property on="Compare String" class="Str"(error in=w372, "DisabledEnum"=w366, "Key Focus"=w364) -> (error out=w371:errorcluster)  [unwired: 1 in, 1 out]
        n164 = call <vilib>:"Add State(s) to Queue__jki_lib_state_machine.vi"("State(s) in (\"\")"=w375) -> ("States Out"=w374:string)  [unwired: 14 in]
      }
      frame "UI: Boolean EnDis" {
        # "Initialize the User Interface, here.\n(this is called automatically, by the Macro: Initialize)"
        n165 = Equal?(x=w382, y="Disable") -> (x = y?=w377:bool)
        n166 = Not(x=w377) -> (.not. x?=w376:bool)
        n167 = Select(t=T6."Disabled and Grayed Out" ("Disabled"), s=w377, f=T6."Enabled" ("Disabled")) -> (s? t:f=w378:T6)
        n168 = property on="Compare Logic" class="CmbBox"(error in=w384, "DisabledEnum"=w378, "Key Focus"=w376) -> (error out=w383:errorcluster)  [unwired: 1 in, 1 out]
        n169 = call <vilib>:"Add State(s) to Queue__jki_lib_state_machine.vi"("State(s) in (\"\")"=w387) -> ("States Out"=w386:string)  [unwired: 14 in]
      }
      frame "UI: Uninitialize" {
        # "Cleanup the User Interface, here.\n(this is called automatically, by the Macro: Exit)"
        n170 = call <vilib>:"Add State(s) to Queue__jki_lib_state_machine.vi"("State(s) in (\"\")"=w391) -> ("States Out"=w390:string)  [unwired: 14 in]
      }
      frame "UI: Cursor Set" {
        # "Argument"
        # "Set and Unset Cursor Busy.\n(Usage: \"UI: Cursor Set >> Busy|Idle\")"
        n171 = case shown="\"Idle\", Default" w392 {
          tunnel: w394 -> [w399 w401]
          tunnel: [w398 w400] -> w393
          frame "Idle", Default {
            n172 = call <vilib>:"Unset Busy.vi"("error in (no error)"=w399) -> ("error out"=w398:errorcluster)  [unwired: 10 in]
          }
          frame "Busy" {
            n173 = call <vilib>:"Set Busy.vi"("error in (no error)"=w401) -> ("error out"=w400:errorcluster)  [unwired: 9 in, 1 out]
          }
        }
        n174 = call <vilib>:"Add State(s) to Queue__jki_lib_state_machine.vi"("State(s) in (\"\")"=w397) -> ("States Out"=w396:string)  [unwired: 14 in]
      }
      frame "UI: Front Panel State" {
        # "Argument"
        # "Set Front Panel Open or Closed\n(Usage: \"UI: Front Panel State >> Open|Close\")"
        n175 = Unbundle By Name(w404) -> ("Core.Current VI Reference"=w403:refnum<vi>)
        n176 = case shown="\"Open\", \"Standard\", Default" w402 {
          tunnel: w406 -> [w414 w429 w440 w453 w466]
          tunnel: [w416 w430 w442 w455 w468] -> w405
          tunnel: w403 -> [w415 w427 w441 w454 w467]
          frame "Open", "Standard", Default {
            w409 = T4."Standard" ("State")
            n177 = property class="VI"(reference=w415, error in=w414) -> (reference out=w412:refnum<vi>, error out=w413:errorcluster, "FP.State"=w411:T4)
            n178 = Not Equal?(x=w411, y=w409) -> (x != y?=w410:bool)
            n179 = case shown="False" w410 {
              tunnel: [w420 w422] -> w416
              tunnel: w413 -> [w419 w422]
              tunnel: w412 -> [w418 _]
              tunnel: w409 -> [w417 _]
              frame True {
                n180 = invoke class="VI" method="FP.Open"(reference=w418, error in=w419, "Activate"=TRUE, "State"=w417) -> (error out=w420:errorcluster)  [unwired: 1 in, 4 out]
              }
              frame False {
              }
            }
          }
          frame "Close", "Closed" {
            n181 = property class="VI"(reference=w427, error in=w429) -> (reference out=w426:refnum<vi>, error out=w428:errorcluster, "FP.State"=w424:T4)
            n182 = Not Equal?(x=w424, y=T4."Closed" ("Front Panel Window:State")) -> (x != y?=w423:bool)
            n183 = case shown="True" w423 {
              tunnel: [w431 w434] -> w430
              tunnel: w428 -> [w431 w433]
              tunnel: w426 -> [_ w432]
              frame False {
              }
              frame True {
                n184 = invoke class="VI" method="FP.Close"(reference=w432, error in=w433) -> (error out=w434:errorcluster)  [unwired: 1 in, 2 out]
              }
            }
          }
          frame "Hidden", "Hide" {
            w435 = T4."Hidden" ("State")
            n185 = property class="VI"(reference=w441, error in=w440) -> (reference out=w438:refnum<vi>, error out=w439:errorcluster, "FP.State"=w437:T4)
            n186 = Not Equal?(x=w437, y=w435) -> (x != y?=w436:bool)
            n187 = case shown="True" w436 {
              tunnel: [w446 w447] -> w442
              tunnel: w439 -> [w445 w447]
              tunnel: w438 -> [w444 _]
              tunnel: w435 -> [w443 _]
              frame True {
                n188 = invoke class="VI" method="FP.Open"(reference=w444, error in=w445, "State"=w443) -> (error out=w446:errorcluster)  [unwired: 2 in, 4 out]
              }
              frame False {
              }
            }
          }
          frame "Minimize", "Minimized" {
            w448 = T4."Minimized" ("State")
            n189 = property class="VI"(reference=w454, error in=w453) -> (reference out=w451:refnum<vi>, error out=w452:errorcluster, "FP.State"=w450:T4)
            n190 = Not Equal?(x=w450, y=w448) -> (x != y?=w449:bool)
            n191 = case shown="True" w449 {
              tunnel: [w459 w460] -> w455
              tunnel: w452 -> [w458 w460]
              tunnel: w451 -> [w457 _]
              tunnel: w448 -> [w456 _]
              frame True {
                n192 = invoke class="VI" method="FP.Open"(reference=w457, error in=w458, "State"=w456) -> (error out=w459:errorcluster)  [unwired: 2 in, 4 out]
              }
              frame False {
              }
            }
          }
          frame "Maximize", "Maximized" {
            w461 = T4."Maximized" ("State")
            n193 = property class="VI"(reference=w467, error in=w466) -> (reference out=w464:refnum<vi>, error out=w465:errorcluster, "FP.State"=w463:T4)
            n194 = Not Equal?(x=w463, y=w461) -> (x != y?=w462:bool)
            n195 = case shown="True" w462 {
              tunnel: [w472 w473] -> w468
              tunnel: w465 -> [w471 w473]
              tunnel: w464 -> [w470 _]
              tunnel: w461 -> [w469 _]
              frame True {
                n196 = invoke class="VI" method="FP.Open"(reference=w470, error in=w471, "State"=w469) -> (error out=w472:errorcluster)  [unwired: 2 in, 4 out]
              }
              frame False {
              }
            }
          }
        }
        n197 = call <vilib>:"Add State(s) to Queue__jki_lib_state_machine.vi"("State(s) in (\"\")"=w408) -> ("States Out"=w407:string)  [unwired: 14 in]
      }
      frame "---------- Macro ----------" {
        # "Do not put any code in this frame.\n(It is a separator no-op. You can make a copy of this frame to create a new Macro frame)"
        n198 = call <vilib>:"Add State(s) to Queue__jki_lib_state_machine.vi"("State(s) in (\"\")"=w477) -> ("States Out"=w476:string)  [unwired: 14 in]
      }
      frame "Macro: Initialize" {
        w478 = "Data: Initialize\nInitialize Core Data\nUI: Initialize\nUI: Front Panel State >> Open\nLimits File: Read Limits file"  # Data: Initialize Initialize Core Data UI: Initialize UI: Front Panel State >> Open Limits File: Read Limits file
        # "Initialization Macro\n(This is called once, when the VI starts)"
        n199 = call <vilib>:"Add State(s) to Queue__jki_lib_state_machine.vi"("State(s) in Front (\"\")"=w478, "State(s) in (\"\")"=w482) -> ("States Out"=w481:string)  [unwired: 13 in]
      }
      frame "Macro: Exit" {
        # "Exit Macro\n(This is called once, when the VI exits)"
        n200 = Unbundle By Name(w489) -> ("Core.Close Panel on Exit?"=w484:bool)
        n201 = call <vilib>:"Conditional State String__jki_lib_state_machine.vi"("Do State(s)?"=w484, "State"="UI: Front Panel State >> Close") -> ("State Out"=w483:string)  [unwired: 7 in]
        n202 = call <vilib>:"Add State(s) to Queue__jki_lib_state_machine.vi"("State(s) in (\"\")"=w483, "State(s) at Back (\"\")"="UI: Uninitialize\nData: Cleanup\nExit") -> ("States Out"=w487:string)  [unwired: 13 in]
        n203 = call <vilib>:"Add State(s) to Queue__jki_lib_state_machine.vi"("State(s) in Front (\"\")"=w487, "State(s) in (\"\")"=w491) -> ("States Out"=w490:string)  [unwired: 13 in]
      }
      frame "---------- Limits File ----------" {
        # "Template Separator\n(You can make a copy of, or modify, this frame)"
        n204 = call <vilib>:"Add State(s) to Queue__jki_lib_state_machine.vi"("State(s) in (\"\")"=w495) -> ("States Out"=w494:string)  [unwired: 14 in]
      }
      frame "Limits File: Read Limits file" {
        w497 = TRUE  # transpose? (F)
        w500 = ","  # delimiter (\t)
        n205 = Unbundle By Name(w499) -> ("Limit File Path"=w498:path)
        n206 = call-poly <vilib>:"Read Delimited Spreadsheet.vi"("file path (dialog if empty)"=w498, "error in (no error)"=w503, "transpose? (F)"=w497, "delimiter (\\t)"=w500) -> ("all rows"=w496:string[][], "error out"=w502:errorcluster)  [unwired: 6 in, 4 out]
        n207 = Bundle By Name(cluster=w499, "Limit File Array"=w496) -> (w501:T7)
        n208 = call <vilib>:"Add State(s) to Queue__jki_lib_state_machine.vi"("State(s) in (\"\")"=w505) -> ("States Out"=w504:string)  [unwired: 14 in]
      }
      frame "Limits File: Build Limits file" {
        n209 = Unbundle By Name(w512) -> ("Test Case"=w508:string, "Limit File Array"=w513:string[][], "Limit Row Array"=w509:string[])
        n210 = Index Array(array=w513) -> (element=w516:string[])  [unwired: 2 in]
        n211 = Insert Into Array(array=w509, index=0, new element=w508) -> (w506:string[])
        n212 = for {
          tunnel: w516 -> [w526] mode=indexing
          tunnel: w508 -> [w525]
          shift-right: [w523] -> _
          shift-left: FALSE -> [w524]
          tunnel: [w520] -> w514
          i -> [w521]
          stop <- w522 stop-if-true
          n213 = case shown="False" w524 {
            selector: w524 -> [_ w534]
            tunnel: w526 -> [w532 w536]
            tunnel: w525 -> [w531 w537]
            tunnel: [w530 w534] -> w523
            tunnel: [FALSE w535] -> w522
            tunnel: w521 -> [w528 w533]
            tunnel: [w527 w533] -> w520
            frame False {
              n214 = Equal?(x=w531, y=w532) -> (x = y?=w530:bool)
              n215 = Increment(x=w528) -> (x+1=w527:i32)
            }
            frame True {
              n216 = Not Equal?(x=w537, y=w536) -> (x != y?=w535:bool)
            }
          }
        }
        n217 = Insert Into Array(array=w513, index (col)=w514, new element=w506) -> (w510:string[][])  [unwired: 1 in]
        n218 = Bundle By Name(cluster=w512, "Limit File Array"=w510) -> (w511:T7)
        n219 = call <vilib>:"Add State(s) to Queue__jki_lib_state_machine.vi"("State(s) in (\"\")"=w519) -> ("States Out"=w518:string)  [unwired: 14 in]
      }
      frame "Limits File: Write Limits file" {
        n220 = Unbundle By Name(w544) -> ("Limit File Path"=w541:path, "Limit File Array"=w540:string[][])
        n221 = call-poly <vilib>:"Write Delimited Spreadsheet.vi"("file path (dialog if empty)"=w541, "2D data"=w540, "error in (no error)"=w542, "transpose? (no:F)"=TRUE, "delimiter (\\t)"="," ("delimiter (\\t)")) -> ("error out"=w543:errorcluster)  [unwired: 9 in, 1 out]
        n222 = call <vilib>:"Add State(s) to Queue__jki_lib_state_machine.vi"("State(s) in (\"\")"=w546) -> ("States Out"=w545:string)  [unwired: 14 in]
      }
    }
  }
  "error out" <- w1
